vi "Lifting.vi"(0 "Direction":enum16{"stop", "up", "down"}(ring), 2 "Down Speed":dbl format="%#_13g", 3 "Mode":enum8{"Start", "Run", "Finish"}(ring), 4 "Up Speed":dbl=0.9 format="%#_13g") -> ()   [LabVIEW 2014]
uses:
  <vilib>/Rock Robotics/SystemInterfaces/DIO/FPGA_DIOPWMChannel.ctl
  <vilib>/Rock Robotics/WPI/MotorControl/WPI_MotorControlOpen Talon.vi
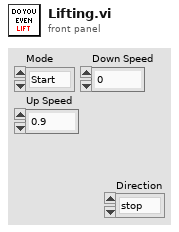
[diagram p1: front panel]
types:
  T1 = typedef "FPGA_DIOPWMChannel.ctl" = enum8{"PWM 0", "PWM 1", "PWM 2", "PWM 3", "PWM 4", "PWM 5", "PWM 6", "PWM 7", "PWM 8", "PWM 9", "PWM MXP 0", "PWM MXP 1", "PWM MXP 2", "PWM MXP 3", "PWM MXP 4", "PWM MXP 5", "PWM MXP 6", "PWM MXP 7", "PWM MXP 8", "PWM MXP 9", "Invalid"}
  T2 = typedef "WPI_MotorControlDeviceRef.ctl" = cluster{"DeviceStatus":errorcluster, "Type":T3, "PWM":cluster{"Controller":T4, "PWM Channel":T1, "DeadBand":T5}, "CAN":cluster{"Device Number":u8, "Control Mode":T6, "Semaphore":T7, "Max Vout":dbl, "TalonSRX Control Mode":T8}, "Invert":bool, "TransformRef":T9, "InvTransformRef":T9}
  T3 = typedef "WPI_MotorControlType.ctl" = enum16{"PWM", "CAN", "CANTalonSRX"}
  T4 = typedef "FPGA_TypedefDigitalModule.ctl" = enum16{"Controller 1"}
  T5 = typedef "WPI_PWMDeadband.ctl" = cluster{"Name":string, "maxPositivePwm":i32, "minPositivePwm":i32, "centerPwm":i32, "maxNegativePwm":i32, "minNegativePwm":i32, "angularRange":u16}
  T6 = typedef "WPI_CANJaguar_ControlMode.ctl" = enum8{"Percent VBus", "Current", "Speed", "Position", "Voltage"}
  T7 = typedef "Semaphore RefNum" = refnum<k1>
  T8 = typedef "WPI_CANTalonSRX_APIControlMode.ctl" = enum8{"Percent VBus", "Speed", "Position", "Slave", "Unchanged / Invalid"}
  T9 = typedef "WPI_PWMTransform_ConPane.ctl" = refnum<vi>
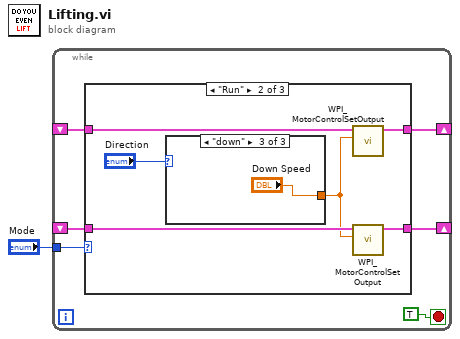
[diagram p0: block diagram]
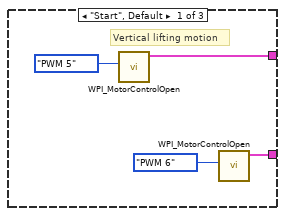
[diagram p2: hidden frame]
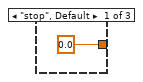
[diagram p3: hidden frame]
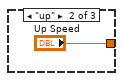
[diagram p4: hidden frame]
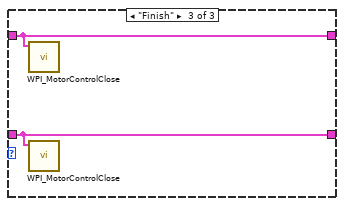
[diagram p5: hidden frame]
diagram:
  n1 = while {
    tunnel: "Mode" -> [w6]
    shift-right: [w5] -> _
    shift-left: _ -> [w3]
    shift-right: [w4] -> _
    shift-left: _ -> [w2]
    stop <- TRUE stop-if-true
    n2 = case shown="\"Run\"" w6 {
      tunnel: [w9 w16 w22] -> w5
      tunnel: [w8 w15 w21] -> w4
      tunnel: w3 -> [_ w17 w22]
      tunnel: w2 -> [_ w14 w21]
      frame "Start", Default {
        # "Vertical lifting motion"
        n3 = call-poly <vilib>:"WPI_MotorControlOpen.vi"("PWM Channel"=FPGA_DIOPWMChannel."PWM 5") -> ("MotorControlDeviceRef"=w9:T2)  [unwired: 9 in, 1 out]
        n4 = call-poly <vilib>:"WPI_MotorControlOpen.vi"("PWM Channel"=FPGA_DIOPWMChannel."PWM 6") -> ("MotorControlDeviceRef"=w8:T2)  [unwired: 9 in, 1 out]
      }
      frame "Run" {
        n5 = case shown="\"down\"" "Direction" {
          tunnel: [0.0 ("downSpeed") "Up Speed" "Down Speed"] -> w12
          frame "stop", Default {
          }
          frame "up" {
          }
          frame "down" {
          }
        }
        n6 = call <vilib>:"WPI_MotorControlSetOutput.vi"("Output"=w12, "MotorControlDevRef"=w17) -> ("MotorControlDevRef"=w16:T2)  [unwired: 7 in, 2 out]
        n7 = call <vilib>:"WPI_MotorControlSetOutput.vi"("Output"=w12, "MotorControlDevRef"=w14) -> ("MotorControlDevRef"=w15:T2)  [unwired: 7 in, 2 out]
      }
      frame "Finish" {
        n8 = call <vilib>:"WPI_MotorControlClose.vi"("MotorControlDevRef"=w22) -> ()  [unwired: 10 in, 1 out]
        n9 = call <vilib>:"WPI_MotorControlClose.vi"("MotorControlDevRef"=w21) -> ()  [unwired: 10 in, 1 out]
      }
    }
  }
